vi "XML ( Clone and Append Multiple Inputs ).vi"(8 "error in (no error)":errorcluster, 9 "Parent_Node":string[](array[string]), 10 "Clone_Node":string[](array[string]), 11 "XML in":refnum<class "XML.lvclass">) -> (0 "error out":errorcluster, 3 "XML out":refnum<class "XML.lvclass">)   [LabVIEW 2018, in "XML.lvlib" / "XML.lvclass"]
uses:
  XML.lvclass
  XML.lvclass/XML.ctl
  <vilib>/xml/Close Reference(Node).vi
  <vilib>/xml/NI_XML.lvlib
  <resource>/objmgr/DOMUserDefRef.rc
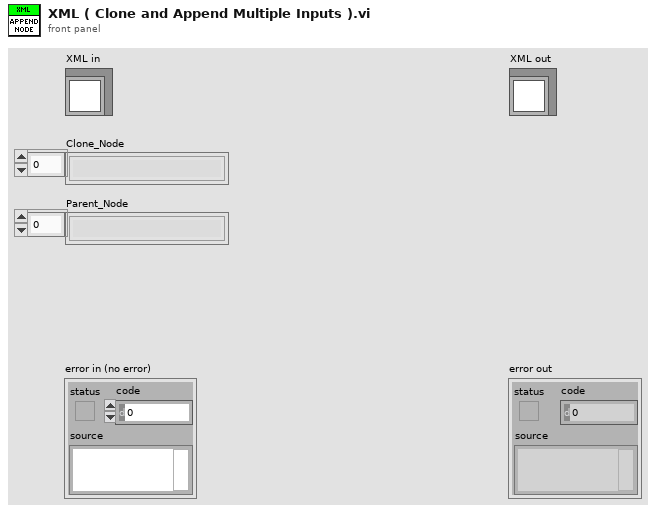
[diagram p1: front panel]
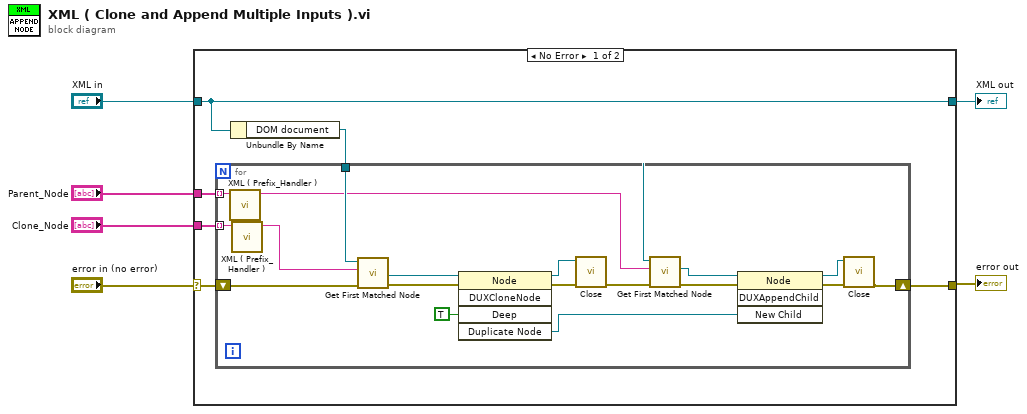
[diagram p0: block diagram]
diagram:
  n1 = case shown="No Error" "error in (no error)" {
    selector: "error in (no error)" -> [w10 w32]
    tunnel: [w9 w32] -> w5
    tunnel: [w12 w31] -> w3
    tunnel: "XML in" -> [w12 w31]
    tunnel: "Clone_Node" -> [w11 _]
    tunnel: "Parent_Node" -> [w7 _]
    frame No Error {
      n2 = Unbundle By Name(w12) -> ("DOM document"=w8:refnum<k20>)
      n3 = for {
        tunnel: w11 -> [w30] mode=indexing
        tunnel: w8 -> [w16]
        tunnel: w7 -> [w15] mode=indexing
        shift-right: [w17] -> w9
        shift-left: w10 -> [w26]
        n4 = call "XML ( Prefix_Handler ).vi"("input string"=w15) -> ("result string"=w14:string)  [unwired: 10 in]
        n5 = call "XML ( Prefix_Handler ).vi"("input string"=w30) -> ("result string"=w13:string)  [unwired: 10 in]
        n6 = call <vilib>:"Get First Matched Node.vi"("error in (no error)"=w26, "XPath expression"=w13, "node in"=w16) -> ("error out"=w25:errorcluster, "node result"=w29:refnum<k20>)  [unwired: 6 in, 1 out]
        n7 = invoke class="Node" method="DUXCloneNode"(reference=w29, error in=w25, "Deep"=TRUE) -> (reference out=w23:refnum<k20>, error out=w24:errorcluster, "Duplicate Node"=w21:refnum<k20>)  [unwired: 2 in, 2 out]
        n8 = call-poly <vilib>:"Close.vi"("error in (no error)"=w24, "node"=w23) -> ("error out"=w20:errorcluster)  [unwired: 7 in]
        n9 = call <vilib>:"Get First Matched Node.vi"("error in (no error)"=w20, "XPath expression"=w14, "node in"=w16) -> ("error out"=w27:errorcluster, "node result"=w22:refnum<k20>)  [unwired: 6 in, 1 out]
        n10 = invoke class="Node" method="DUXAppendChild"(reference=w22, error in=w27, "New Child"=w21) -> (reference out=w18:refnum<k20>, error out=w19:errorcluster)  [unwired: 1 in, 2 out]
        n11 = call-poly <vilib>:"Close.vi"("error in (no error)"=w19, "node"=w18) -> ("error out"=w17:errorcluster)  [unwired: 7 in]
      }
    }
    frame Error {
    }
  }
  "error out" <- w5
  "XML out" <- w3
